vi "12x12 Mapping Data Read.vi"(8 "error constant":errorcluster, 10 "Small File name":string="QS", 11 "Path":path=path "E:/Documents/lab") -> (0 "error out":errorcluster, 2 "all rows":dbl[][][][](array[numeric]))   [LabVIEW 2012]
doc: "This VI Takes a two letter name (QS) and finds 36 files named E:\\Documents\\lab\\QS\\OQS##LE.DAT\nwhere ## are [A,F][A,F]. It then builds a 4D array:\n1 X position on sample (0-5 for [A,F])\n2 Y position on sample (same as above)\n3 index of array (0- 511 one for each pixel)\n4 Rcm-1 and Counts at that index (0 or 1)"
uses:
  <vilib>/Utility/file.llb/Read From Spreadsheet File (DBL).vi
panel:
  out "XY Graph":cluster{"Y":dbl[], "Y":dbl[]}[](graph)
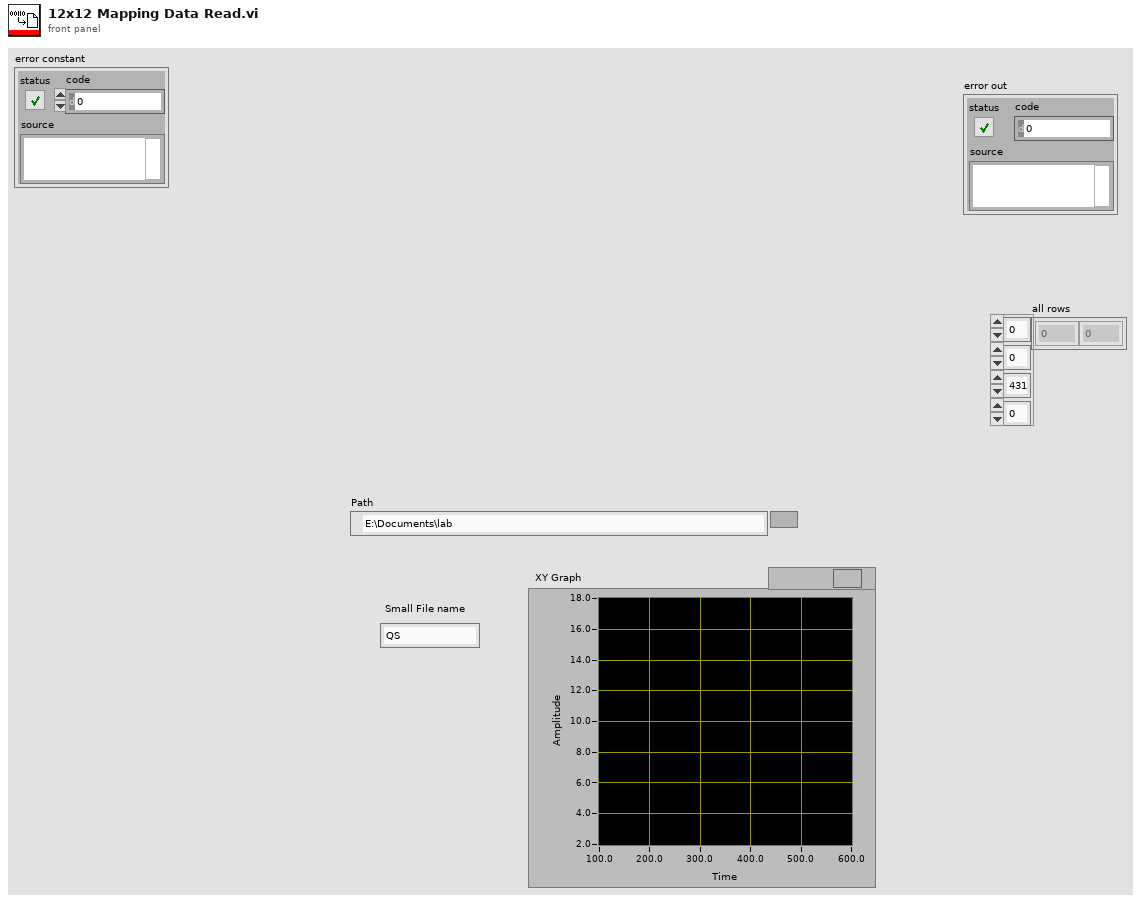
[diagram p1: front panel]
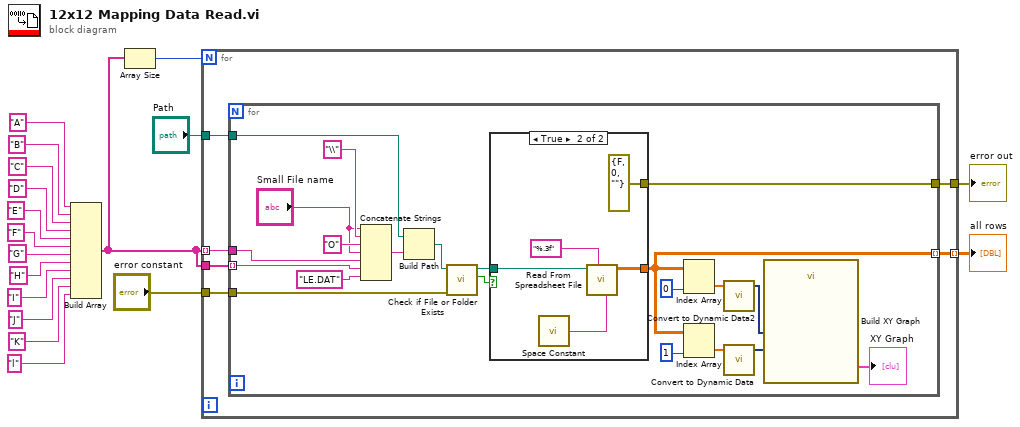
[diagram p0: block diagram]
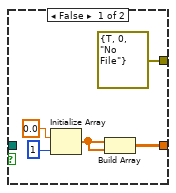
[diagram p2: hidden frame]
diagram:
  n1 = Build Array("A", "B", "C", "D", "E", "F", "G" ("element"), "H" ("element"), "I" ("element"), "J" ("element"), "K" ("element"), "l" ("element")) -> (w11:string[])
  n2 = Array Size(array=w11) -> (size(s)=w18:i32)
  n3 = for {
    N: w18 -> [_]
    tunnel: w11 -> [w24]
    tunnel: w11 -> [w23] mode=indexing
    tunnel: "Path" -> [w22]
    tunnel: [w21] -> w9 mode=indexing
    tunnel: "error constant" -> [w20]
    tunnel: [w19] -> w7
    n4 = for {
      tunnel: w24 -> [w35] mode=indexing
      tunnel: w23 -> [w34]
      tunnel: w22 -> [w31]
      tunnel: [w28] -> w21 mode=indexing
      tunnel: w20 -> [w26]
      tunnel: [w25] -> w19
      n5 = Concatenate Strings("Small File name", "\\", "O", "Small File name", w34, w35, "LE.DAT") -> (w32:string)
      n6 = Build Path(base path=w31, name or relative path=w32) -> (appended path=w30:path)
      n7 = call <vilib>:"Check if File or Folder Exists.vi"("error in (no error)"=w26, "path"=w30) -> ("file or folder exists?"=w29:bool, "dup path"=w27:path)  [unwired: 7 in, 1 out]
      n8 = case shown="True" w29 {
        tunnel: [w47 w53] -> w28
        tunnel: w27 -> [_ w52]
        tunnel: [errorcluster {"status"=TRUE, "code"=0, "source"="No File"} ("error constant") errorcluster {"status"=FALSE, "code"=0, "source"=""} ("error constant")] -> w25
        frame False {
          n9 = Initialize Array(0.0 ("element"), 1 ("dimension size")) -> (w48:dbl[])
          n10 = Build Array(w48, w48) -> (w47:dbl[][])
        }
        frame True {
          n11 = call <vilib>:"Space Constant.vi"() -> ("String"=w54:string)
          n12 = call-poly <vilib>:"Read From Spreadsheet File.vi"("delimiter (\\t)"=w54, "format (%.3f)"="%.3f", "file path (dialog if empty)"=w52) -> ("all rows"=w53:dbl[][])  [unwired: 4 in, 4 out]
        }
      }
      n13 = Index Array(array=w28, index (col)=0 ("index (row)")) -> (element=w42:dbl[])  [unwired: 1 in]
      n14 = Index Array(array=w28, index (col)=1 ("index (row)")) -> (element=w40:dbl[])  [unwired: 1 in]
      n15 = call "Convert to Dynamic Data2"("Array"=w42) -> ("Dynamic Data Type"=w43:dynamicdata)  [unwired: 3 in]
      n16 = call "Convert to Dynamic Data"("Array"=w40) -> ("Dynamic Data Type"=w41:dynamicdata)  [unwired: 3 in]
      n17 = call "Build XY Graph"("Y Input"=w41, "X Input"=w43) -> ("XY Graph"=→"XY Graph":cluster{"Y":dbl[], "Y":dbl[]}[])  [unwired: 3 in, 6 out]
    }
  }
  "all rows" <- w9
  "error out" <- w7
